vi "Acquire_OSCILL_SubVI.vi"(8 "error in (no error)":errorcluster, 9 "Vertical Scale[mV]":dbl=5.0, 10 "N_acquisition":i32, 11 "VISA resource name":refnum<visa-resource-name>) -> (0 "error out":errorcluster, 1 "Time":dbl[](array[numeric]), 2 "CH2_averaged":dbl[](array[numeric]), 3 "CH1_averaged":dbl[](array[numeric]), 5 "VISA resource name out":refnum<visa-resource-name>)   [LabVIEW 2017]
uses:
  Agilent 2000 3000 X-Series/Agilent 2000 3000 X-Series.lvlib
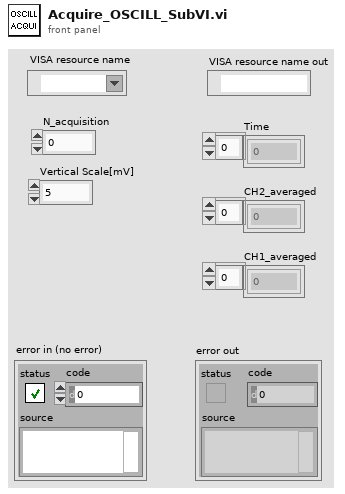
[diagram p1: front panel]
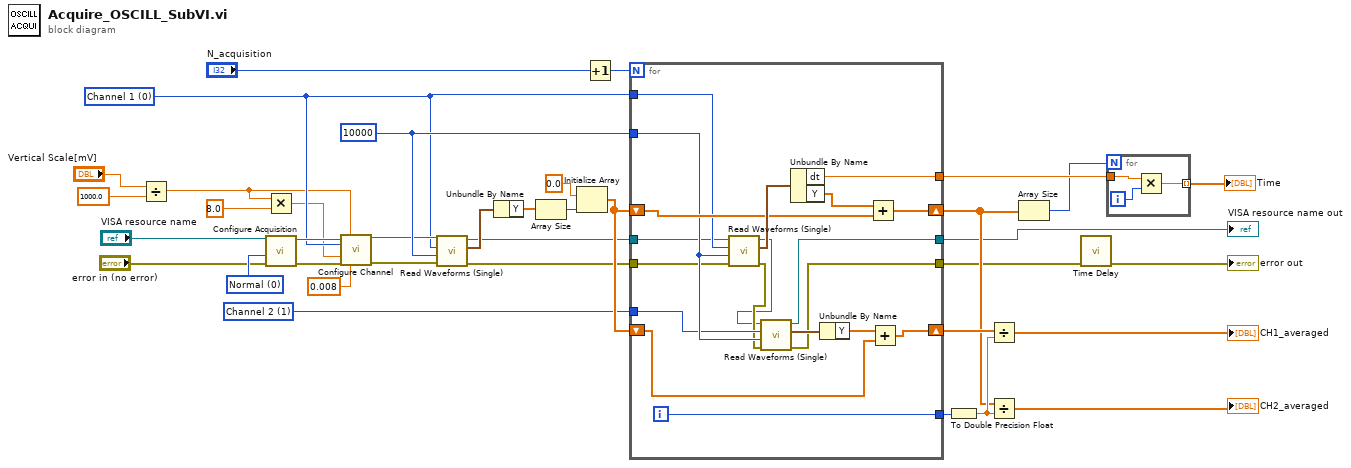
[diagram p0: block diagram]
diagram:
  w33 = 1 items=["Channel 1"=0, "Channel 2"=1, "Channel 3"=2, "Channel 4"=3, "Digital Bus Low"=9, "Digital Bus High"=10] ("Source Channel (0: Channel 1)")
  w16 = 0 items=["Channel 1"=0, "Channel 2"=1, "Channel 3"=2, "Channel 4"=3, "Digital Bus Low"=9, "Digital Bus High"=10] ("Source Channel (0: Channel 1)")
  w31 = 0 items=["Normal", "Average", "High Resolution", "Peak"] ("Acquisition Type (0: Normal)")
  w32 = u32 10000 ("y")
  n1 = Divide(x="Vertical Scale[mV]", y=1000.0) -> (x/y=w12:dbl)
  n2 = Multiply(x=w12, y=8.0) -> (x*y=w13:dbl)
  n3 = call "Configure Acquisition.vi"("error in (no error)"="error in (no error)", "Acquisition Type (0: Normal)"=w31, "VISA resource name"="VISA resource name") -> ("error out"=w17:errorcluster, "VISA resource name out"=w18:refnum<visa-resource-name>)  [unwired: 7 in]
  n4 = call "Configure Channel.vi"("VISA resource name"=w18, "Vertical Scale (5.0 V)"=w12, "Channel Name (0: Channel 1)"=w16, "Vertical Range (40.0 V)"=w13, "error in (no error)"=w17, "Vertical Offset (0.0)"=0.008) -> ("VISA resource name out"=w20:refnum<visa-resource-name>, "error out"=w19:errorcluster)  [unwired: 5 in, 3 out]
  n5 = call "Read Waveforms (Single).vi"("error in (no error)"=w19, "Timeout (10000 ms)"=w32, "Source Channel (0: Channel 1)"=w16, "VISA resource name"=w20) -> ("error out"=w8:errorcluster, "Waveform Data"=w28:waveform(dbl), "VISA resource name out"=w7:refnum<visa-resource-name>)  [unwired: 1 in, 4 out]
  n6 = Unbundle By Name(w28) -> ("Y"=w29:dbl[])
  n7 = Array Size(array=w29) -> (size(s)=w30:i32)
  n8 = Initialize Array(0.0 ("element"), w30) -> (w35:dbl[])
  n9 = Increment(x="N_acquisition") -> (x+1=w24:i32)
  n10 = for {
    N: w24 -> [_]
    tunnel: w32 -> [w49]
    tunnel: w16 -> [w50]
    tunnel: [w55] -> w22
    shift-right: [w52] -> w26
    shift-left: w35 -> [w54]
    tunnel: [w53] -> w25
    tunnel: w33 -> [w48]
    shift-right: [w45] -> w37
    shift-left: w35 -> [w44]
    tunnel: w8 -> [w41]
    tunnel: w7 -> [w40]
    tunnel: [w39] -> w6
    tunnel: [w38] -> w1
    i -> [w53]
    n11 = call "Read Waveforms (Single).vi"("error in (no error)"=w41, "Timeout (10000 ms)"=w49, "Source Channel (0: Channel 1)"=w50, "VISA resource name"=w40) -> ("error out"=w43:errorcluster, "Waveform Data"=w56:waveform(dbl), "VISA resource name out"=w42:refnum<visa-resource-name>)  [unwired: 1 in, 4 out]
    n12 = call "Read Waveforms (Single).vi"("error in (no error)"=w43, "Timeout (10000 ms)"=w49, "Source Channel (0: Channel 1)"=w48, "VISA resource name"=w42) -> ("error out"=w38:errorcluster, "Waveform Data"=w47:waveform(dbl), "VISA resource name out"=w39:refnum<visa-resource-name>)  [unwired: 1 in, 4 out]
    n13 = Unbundle By Name(w56) -> ("dt"=w55:dbl, "Y"=w51:dbl[])
    n14 = Unbundle By Name(w47) -> ("Y"=w46:dbl[])
    n15 = Add(x=w51, y=w54) -> (x+y=w52:dbl[])
    n16 = Add(x=w46, y=w44) -> (x+y=w45:dbl[])
  }
  "VISA resource name out" <- w6
  n17 = To Double Precision Float(number=w25) -> (double precision float=w36:dbl)
  n18 = Divide(x=w37, y=w36) -> (x/y=→"CH1_averaged":dbl[])
  n19 = Divide(x=w26, y=w36) -> (x/y=→"CH2_averaged":dbl[])
  n20 = Array Size(array=w26) -> (size(s)=w21:i32)
  n21 = call "Time Delay"("error in (no error)"=w1) -> ("error out"=→"error out":errorcluster)  [unwired: 10 in]
  n22 = for {
    N: w21 -> [_]
    tunnel: w22 -> [w58]
    tunnel: [w59] -> w34 mode=indexing
    i -> [w57]
    n23 = Multiply(x=w58, y=w57) -> (x*y=w59:dbl)
  }
  "Time" <- w34
